vi "Read Configurations.vi"(8 "error in (no error)":errorcluster) -> (0 "error out":errorcluster, 3 "Device Parameters":T1={"Device"=enum."Exec"})   [LabVIEW 2020]
uses:
  Type Definitions/Device Parameters.ctl
  Type Definitions/Device.ctl
  <vilib>/Utility/config.llb/Read Key (String).vi
  <vilib>/Utility/config.llb/NI_LVConfig.lvlib
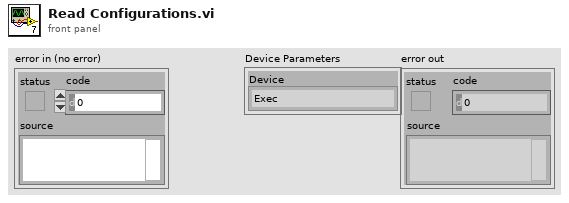
[diagram p1: front panel]
types:
  T1 = typedef "Device Parameters.ctl" = cluster{"Device":T2}
  T2 = typedef "Device.ctl" = enum32{"None", "Exec", "Aux1", "Aux2", "Aux3"}
  T3 = typedef "NI_LVConfig.lvlib/Config Data RefNum.ctl" = refnum<k1>
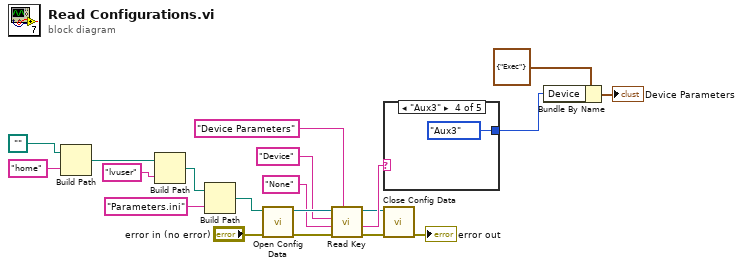
[diagram p0: block diagram]
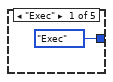
[diagram p2: hidden frame]
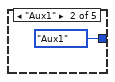
[diagram p3: hidden frame]
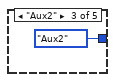
[diagram p4: hidden frame]
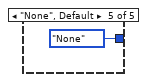
[diagram p5: hidden frame]
diagram:
  n1 = Build Path(base path=path "", name or relative path="home") -> (appended path=w16:path)
  n2 = Build Path(base path=w16, name or relative path="lvuser") -> (appended path=w18:path)
  n3 = Build Path(base path=w18, name or relative path="Parameters.ini") -> (appended path=w20:path)
  n4 = call <vilib>:"Open Config Data.vi"("error in (no error)"="error in (no error)", "configuration file path"=w20) -> ("error out"=w3:errorcluster, "refnum"=w13:T3)  [unwired: 7 in, 1 out]
  n5 = call-poly <vilib>:"Read Key.vi"("section"="Device Parameters", "error in (no error)"=w3, "default value"="None", "key"="Device", "refnum"=w13) -> ("error out"=w2:errorcluster, "value"=w9:string, "refnum out"=w6:T3)  [unwired: 3 in, 1 out]
  n6 = case shown="\"Aux3\"" w9 {
    tunnel: [Device."Exec" ("Device") Device."Aux1" ("Device") Device."Aux2" ("Device") Device."Aux3" ("Device") Device."None" ("Device")] -> w7
    frame "Exec" {
    }
    frame "Aux1" {
    }
    frame "Aux2" {
    }
    frame "Aux3" {
    }
    frame "None", Default {
    }
  }
  n7 = call <vilib>:"Close Config Data.vi"("error in (no error)"=w2, "refnum"=w6) -> ("error out"=→"error out":errorcluster)  [unwired: 8 in, 1 out]
  n8 = Bundle By Name(cluster=T1 {"Device"=enum."Exec"}, "Device"=w7) -> (→"Device Parameters":T1)
